vi "Set StartPoint.vi"(8 "error in (no error)":errorcluster, 10 "StartPoint":cluster{"x":i16, "y":i16}, 11 "Line Border in":refnum<class "Line Border.lvclass">) -> (0 "error out":errorcluster, 3 "Line Border out":refnum<class "Line Border.lvclass">)   [LabVIEW 2015, in "Line Border.lvclass"]
uses:
  Line Border.lvclass
  Line Border.lvclass/Line Border.ctl
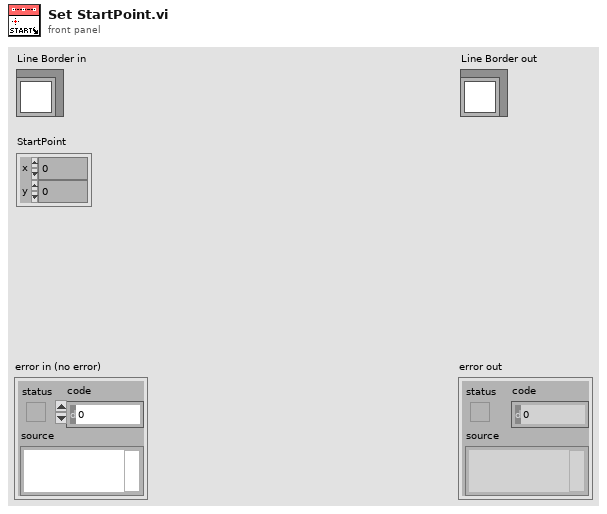
[diagram p1: front panel]
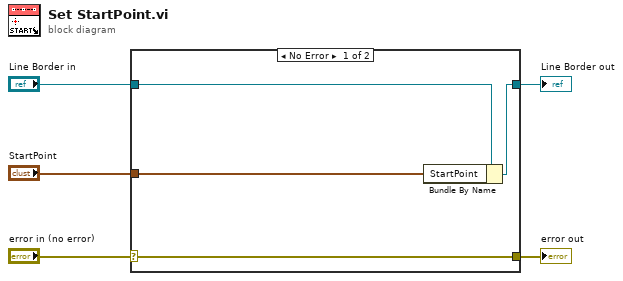
[diagram p0: block diagram]
diagram:
  n1 = case shown="No Error" "error in (no error)" {
    selector: "error in (no error)" -> [w9 w10]
    tunnel: [w9 w10] -> w4
    tunnel: [w7 w11] -> w2
    tunnel: "Line Border in" -> [w8 w11]
    tunnel: "StartPoint" -> [w6 _]
    frame No Error {
      n2 = Bundle By Name(cluster=w8, "StartPoint"=w6) -> (w7:refnum<class "Line Border.lvclass">)
    }
    frame Error {
    }
  }
  "error out" <- w4
  "Line Border out" <- w2
